vi "Open Vi Reference.vi"(2 "error in (no error)":errorcluster, 3 "Show":bool=TRUE, 4 "RunVi":bool, 5 "reference":refnum<vi>) -> (0 "error out":errorcluster, 1 "reference out":refnum<vi>)   [LabVIEW 2011]
panel:
  out "Execution:State":T1(ring)
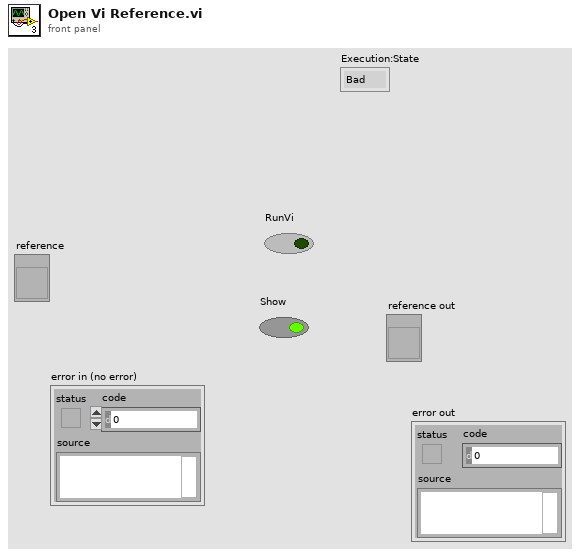
[diagram p1: front panel]
types:
  T1 = enum32{"Bad", "Idle", "Run top level", "Running"}
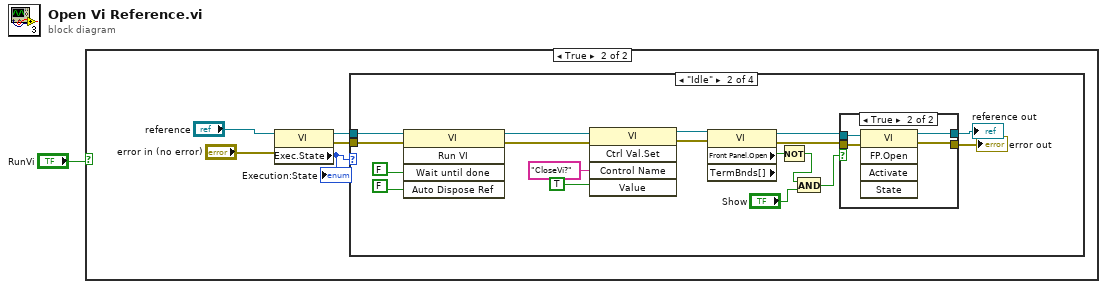
[diagram p0: block diagram]
diagram:
  n1 = case shown="True" "RunVi" {
    frame False {
    }
    frame True {
      n2 = property class="VI"(reference="reference", error in="error in (no error)") -> (reference out=w3:refnum<vi>, error out=w4:errorcluster, "Exec.State"=w2:T1)
      "Execution:State" <- w2
      n3 = case shown="\"Idle\"" w2 {
        tunnel: w4 -> [_ w18 _ _]
        tunnel: w3 -> [_ w17 _ _]
        frame "Bad", Default {
        }
        frame "Idle" {
          n4 = invoke class="VI" method="Run VI"(reference=w17, error in=w18, "Wait until done"=FALSE ("Wait Until Done"), "Auto Dispose Ref"=FALSE ("Auto Dispose Reference")) -> (reference out=w14:refnum<vi>, error out=w13:errorcluster)  [unwired: 1 in, 3 out]
          n5 = invoke class="VI" method="Ctrl Val.Set"(reference=w14, error in=w13, "Control Name"="CloseVi?", "Value"=TRUE ("Auto Dispose Reference")) -> (reference out=w12:refnum<vi>, error out=w11:errorcluster)  [unwired: 1 in, 3 out]
          n6 = property class="VI" props=["Front Panel.Open", "TermBnds[]"](reference=w12, error in=w11) -> (reference out=w21:refnum<vi>, error out=w20:errorcluster, "Front Panel.Open"=w8:bool)  [unwired: 1 out]
          n7 = Not(x=w8) -> (.not. x?=w9:bool)
          n8 = And(x=w9, y="Show") -> (x .and. y?=w7:bool)
          n9 = case shown="True" w7 {
            tunnel: w21 -> [w26 w30]
            tunnel: w20 -> [w25 w29]
            tunnel: [w26 w28] -> w22
            tunnel: [w25 w27] -> w19
            frame False {
            }
            frame True {
              n10 = invoke class="VI" method="FP.Open"(reference=w30, error in=w29) -> (reference out=w28:refnum<vi>, error out=w27:errorcluster)  [unwired: 3 in, 3 out]
            }
          }
          "reference out" <- w22
          "error out" <- w19
        }
        frame "Run top level" {
        }
        frame "Running" {
        }
      }
    }
  }
